vi "Untitled 1.vi"() -> ()   [LabVIEW 2023]
uses:
  <vilib>/numeric/Random Number (Range) I64.vi
  <vilib>/numeric/sub_Random U32.vi
  <vilib>/Utility/file.llb/Read Delimited Spreadsheet (string).vi
  <vilib>/Utility/file.llb/Write Delimited Spreadsheet (string).vi
panel:
  out "all rows":string[][](array[string])
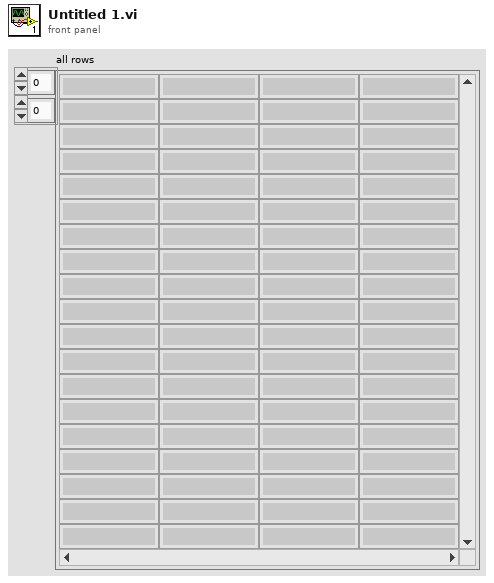
[diagram p1: front panel]
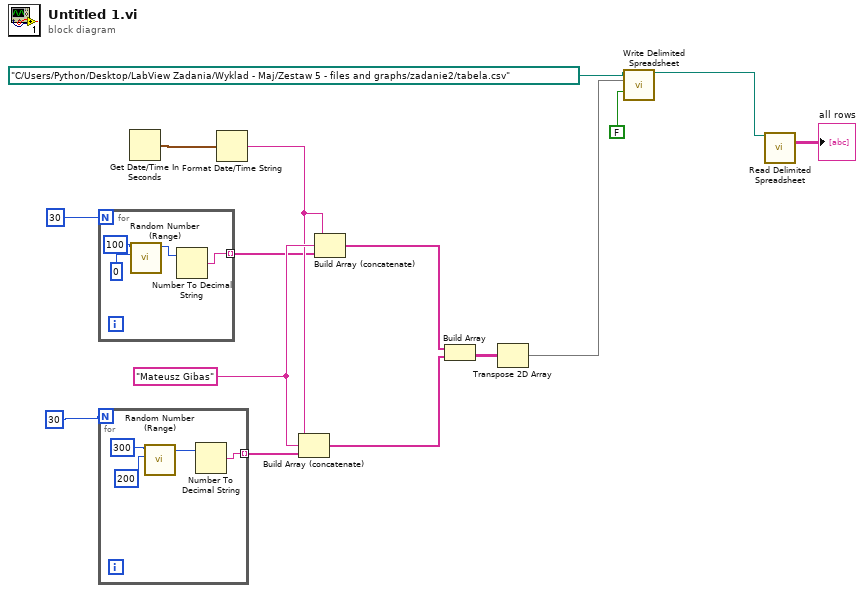
[diagram p0: block diagram]
diagram:
  w10 = "Mateusz Gibas"
  n1 = for {
    N: 30 -> [_]
    tunnel: [w16] -> w7 mode=indexing
    n2 = call-poly <vilib>:"Random Number (Range).vi"("lower bound (-100)"=i64 0, "upper bound (100)"=i64 100) -> ("number"=w17:i64)  [unwired: 9 in]
    n3 = Number To Decimal String(number=w17) -> (decimal integer string=w16:string)  [unwired: 1 in]
  }
  n4 = for {
    N: 30 -> [_]
    tunnel: [w20] -> w8 mode=indexing
    n5 = call-poly <vilib>:"Random Number (Range).vi"("lower bound (-100)"=i64 200, "upper bound (100)"=i64 300) -> ("number"=w21:i64)  [unwired: 9 in]
    n6 = Number To Decimal String(number=w21) -> (decimal integer string=w20:string)  [unwired: 1 in]
  }
  n7 = Get Date/Time In Seconds() -> (seconds since 1Jan1904=w13:timestamp)
  n8 = Format Date/Time String(seconds (now)=w13) -> (date/time string=w9:string)  [unwired: 2 in]
  n9 = Build Array (concatenate)(w9, w10, w8) -> (w12:string[])
  n10 = Build Array (concatenate)(w9, w10, w7) -> (w11:string[])
  n11 = Build Array(w11, w12) -> (w5:string[][])
  n12 = Transpose 2D Array(2D array=w5) -> (transposed array=w4:string[][])
  n13 = call-poly <vilib>:"Write Delimited Spreadsheet.vi"("file path (dialog if empty)"=path "C:/Users/Python/Desktop/LabView Zadania/Wyklad - Maj/Zestaw 5 - files and graphs/zadanie2/tabela.csv", "2D data"=w4, "append to file? (new file:F)"=FALSE) -> ("new file path (Not A Path if cancelled)"=w1:path)  [unwired: 11 in, 1 out]
  n14 = call-poly <vilib>:"Read Delimited Spreadsheet.vi"("file path (dialog if empty)"=w1) -> ("all rows"=→"all rows":string[][])  [unwired: 9 in, 5 out]
